vi "PIDController_Pack_AdvLimits.vi"(4 "MinOutput":dbl=-9.9e+32, 6 "MaxOutput":dbl=9.9e+32, 9 "Continuous":bool, 10 "MinInput":dbl, 11 "MaxInput":dbl) -> (3 "Adv PID Limits":T1={"MaxInput"=0.0, "MinInput"=0.0, "Continuous"=FALSE, "MaxOutput"=9.9e+32, "MinOutput"=-9.9e+32})   [LabVIEW 2019, in "Trajectory_Library.lvlib"]
uses:
  Trajectory_Library.lvlib
  PID_ADV_LIMITS.ctl
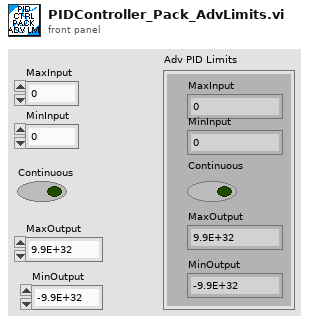
[diagram p1: front panel]
types:
  T1 = typedef "Trajectory_Library.lvlib/PID_ADV_LIMITS.ctl" = cluster{"MaxInput":dbl, "MinInput":dbl, "Continuous":bool, "MaxOutput":dbl, "MinOutput":dbl}
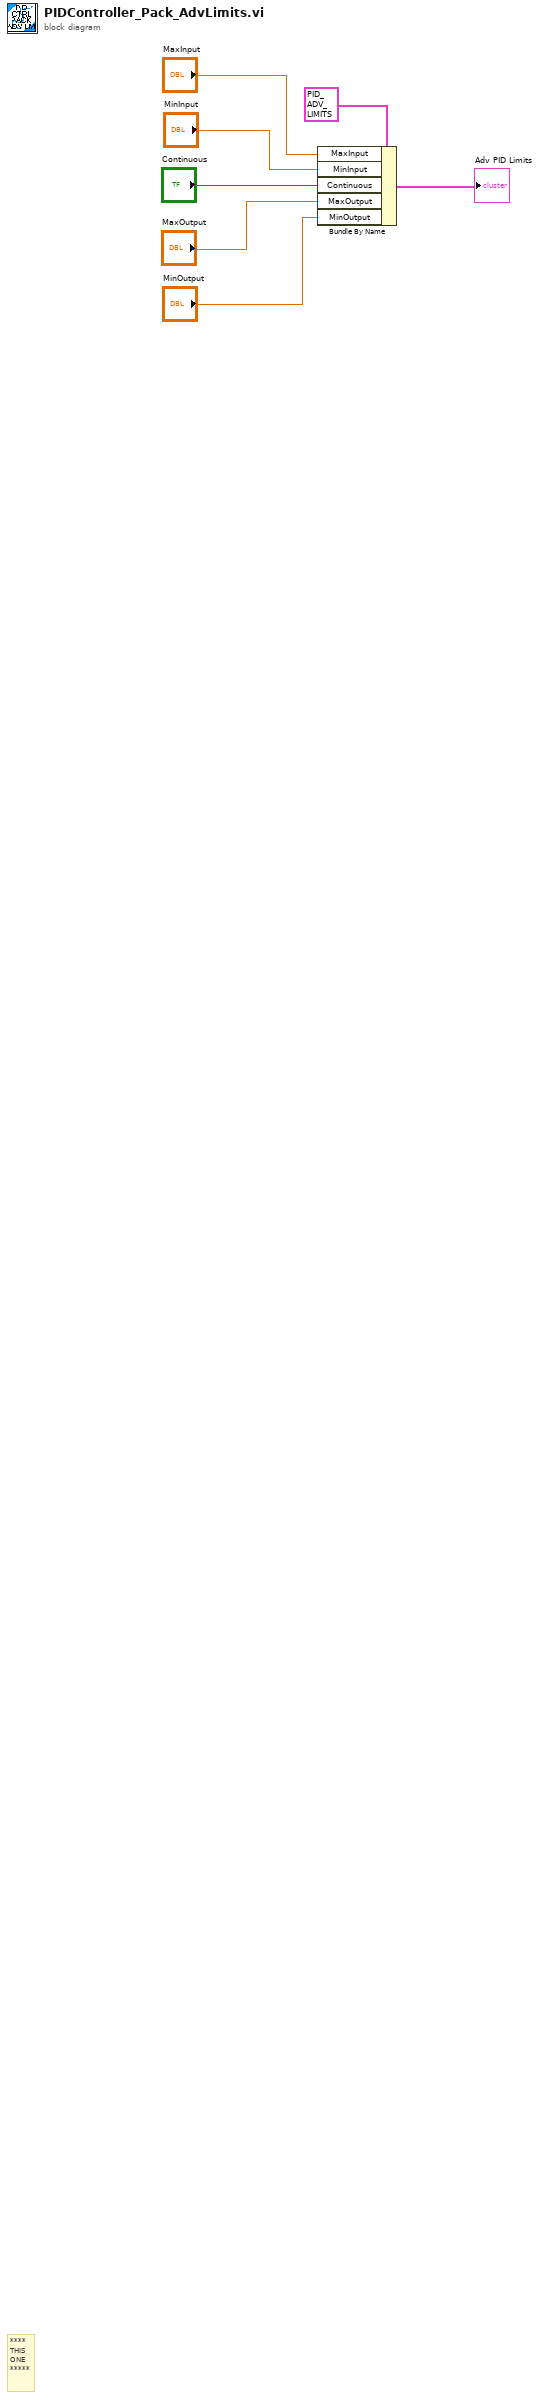
[diagram p0: block diagram]
diagram:
  # "****\nTHIS\nONE\n*****"
  n1 = Bundle By Name(cluster=T1 {"MaxInput"=0.0, "MinInput"=0.0, "Continuous"=FALSE, "MaxOutput"=9.9e+32, "MinOutput"=-9.9e+32} ("Adv PID Limits"), "MaxInput"="MaxInput", "MinInput"="MinInput", "Continuous"="Continuous", "MaxOutput"="MaxOutput", "MinOutput"="MinOutput") -> (→"Adv PID Limits":T1)
